vi "RT Errors.Set Error Code.vi"(10 "code":i32, 11 "error in":errorcluster) -> (3 "error out":errorcluster)   [LabVIEW 2016, in "RT Error Handling.lvlib"]
uses:
  RT Error Handling.lvlib
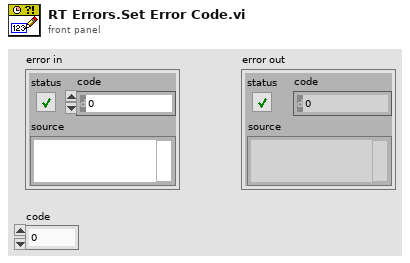
[diagram p1: front panel]
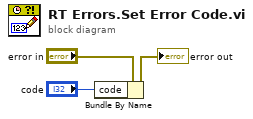
[diagram p0: block diagram]
diagram:
  n1 = Bundle By Name(cluster="error in", "code"="code") -> (→"error out":errorcluster)
